vi "Eat.vi"(8 "error in (no error)":errorcluster, 10 "String":string, 11 "Tiger in":refnum<class "Tiger.lvclass">) -> (0 "error out":errorcluster, 2 "String 2":string, 3 "Tiger out":refnum<class "Tiger.lvclass">)   [LabVIEW 2018, in "Tiger.lvclass"]
uses:
  Tiger.lvclass
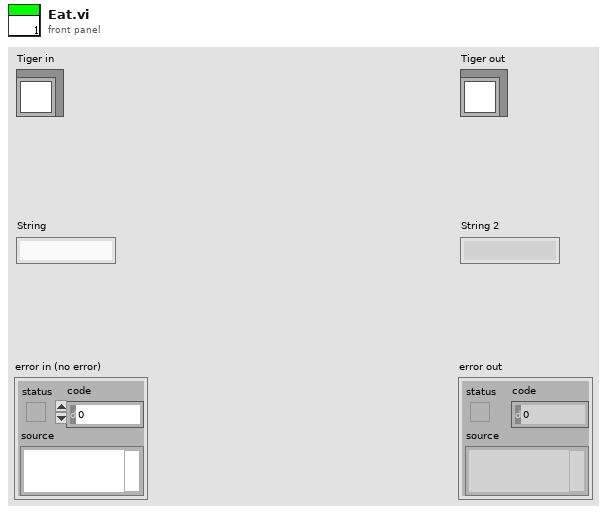
[diagram p1: front panel]
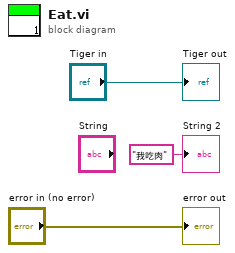
[diagram p0: block diagram]
diagram:
  "error out" <- "error in (no error)"
  "Tiger out" <- "Tiger in"
  "String 2" <- "我吃肉" ("String 2")
